vi "CreateBPMDAQTask.vi"(8 "Error In":errorcluster) -> (0 "Error Out":errorcluster, 3 "BPM Task":refnum<k21>)   [LabVIEW 2012]
uses:
  <vilib>/DAQmx/create/channels.llb/DAQmx Create Channel (AI-Voltage-Basic).vi
  <vilib>/DAQmx/configure/timing.llb/DAQmx Timing (Sample Clock).vi
  <vilib>/DAQmx/configure/trigger.llb/DAQmx Start Trigger (Digital Edge).vi
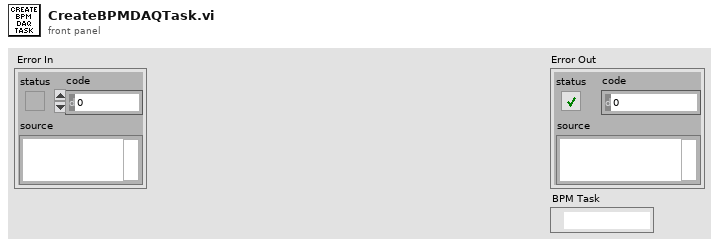
[diagram p1: front panel]
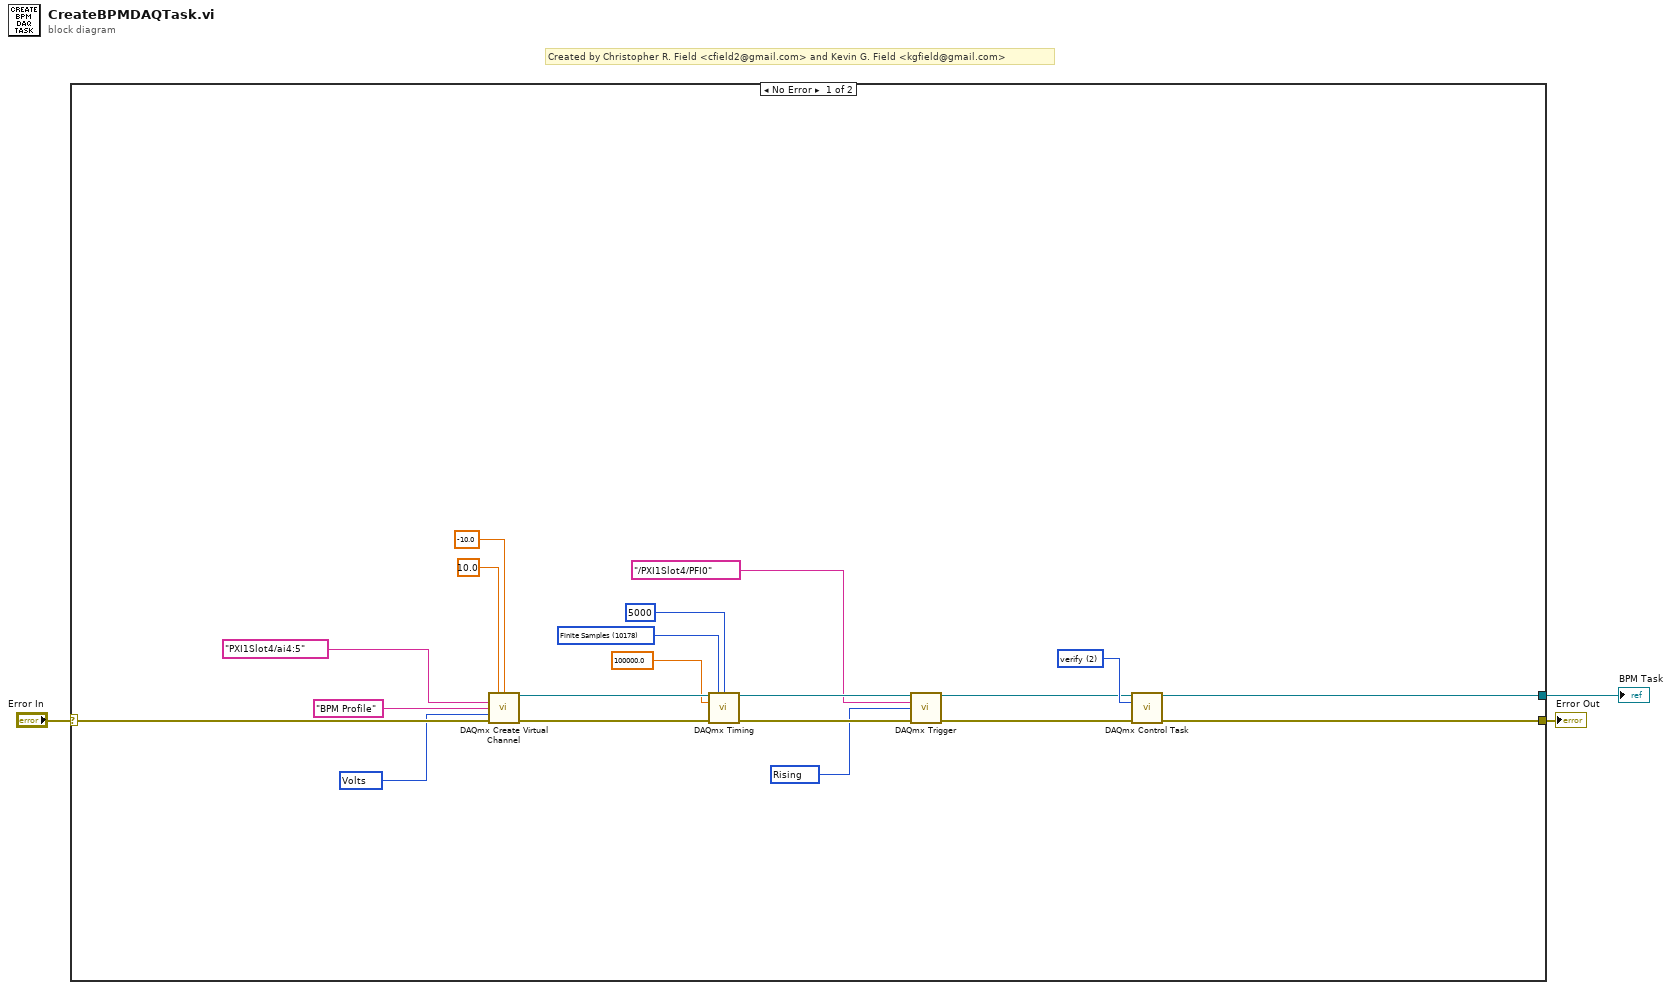
[diagram p0: block diagram]
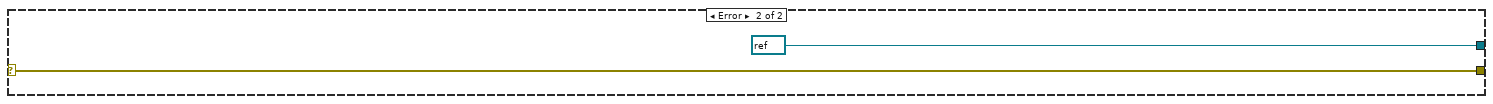
[diagram p2: hidden frame]
diagram:
  # "Created by Christopher R. Field <cfield2@gmail.com> and Kevin G. Field <kgfield@gmail.com>"
  n1 = case shown="No Error" "Error In" {
    selector: "Error In" -> [w23 w25]
    tunnel: [w22 w25] -> w2
    tunnel: [w21 refnum<k21> refnum ("task out")] -> w1
    frame No Error {
      w8 = 10280 items=["Rising"=10280, "Falling"=10171] ("edge")
      w13 = 10348 items=["Volts"=10348, "From Custom Scale"=10065] ("units")
      w14 = 2 items=["verify"=2, "reserve"=4, "commit"=3, "unreserve"=5, "abort"=6] ("action")
      w16 = 10178 items=["Finite Samples"=10178, "Continuous Samples"=10123, "Hardware Timed Single Point"=12522] ("sample mode")
      n2 = call-poly <vilib>:"DAQmx Create Virtual Channel.vi"("maximum value"=10.0, "minimum value"=-10.0, "physical channels"=tag "PXI1Slot4/ai4:5", "name to assign"="BPM Profile", "units"=w13, "error in"=w23) -> ("task out"=w20:refnum<k21>, "error out"=w19:errorcluster)  [unwired: 8 in]
      n3 = call-poly <vilib>:"DAQmx Timing.vi"("task/channels in"=w20, "sample mode"=w16, "samples per channel"=5000, "rate"=100000.0, "error in"=w19) -> ("task out"=w12:refnum<k21>, "error out"=w9:errorcluster)  [unwired: 9 in]
      n4 = call-poly <vilib>:"DAQmx Trigger.vi"("task/channels in"=w12, "source"=tag "/PXI1Slot4/PFI0", "edge"=w8, "error in"=w9) -> ("task out"=w11:refnum<k21>, "error out"=w10:errorcluster)  [unwired: 10 in]
      n5 = call <vilib>:"DAQmx Control Task.vi"("task/channels in"=w11, "action"=w14, "error in"=w10) -> ("task out"=w21:refnum<k21>, "error out"=w22:errorcluster)  [unwired: 11 in]
    }
    frame Error {
    }
  }
  "Error Out" <- w2
  "BPM Task" <- w1
